vi "get data dimensions.vi"(8 "error in":errorcluster, 10 "# of groups":i32, 11 "Data (Dictionary)":T1[](array[typedef])) -> (0 "error out":errorcluster, 3 "data dimensions":i32[](array[numeric]))   [LabVIEW 2016]
uses:
  <userlib>/LevyLab/LV to ITX/Data/Typedefs/Dictionary--cluster.ctl
  <userlib>/LevyLab/LV to ITX/Data/Data.lvclass
panel:
  out "# groups (itx files)":i32
  out "# channels per file":i32
  out "# data pts per channel":dbl
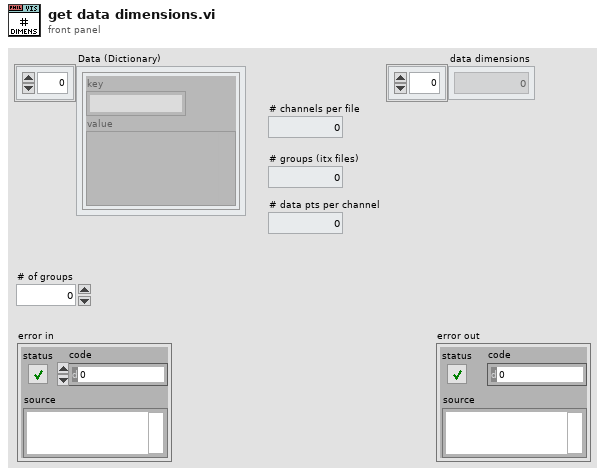
[diagram p1: front panel]
types:
  T1 = typedef "Data.lvclass/Dictionary--cluster.ctl" = cluster{"key":string, "value":variant}
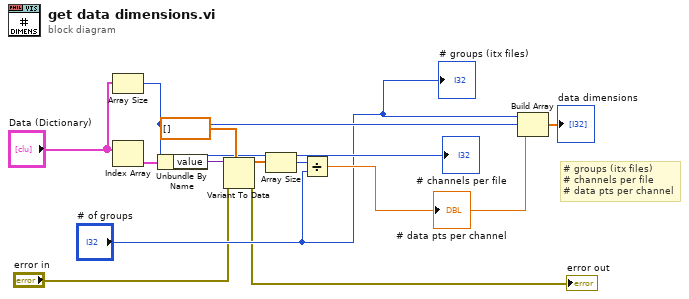
[diagram p0: block diagram]
diagram:
  # "# groups (itx files)\n# channels per file\n# data pts per channel"
  n1 = Array Size(array="Data (Dictionary)") -> (size(s)=w5:i32)
  "# channels per file" <- w5
  n2 = Index Array(array="Data (Dictionary)") -> (element=w8:T1)  [unwired: 1 in]
  n3 = Unbundle By Name(w8) -> ("value"=w9:variant)
  n4 = Variant To Data(error in="error in", type=dbl[] [], Variant=w9) -> (data=w11:dbl[], error out=→"error out":errorcluster)
  n5 = Array Size(array=w11) -> (size(s)=w12:i32)
  n6 = Divide(x=w12, y="# of groups") -> (x/y=w6:dbl)
  "# data pts per channel" <- w6
  n7 = Build Array("# of groups", w5, w6) -> (→"data dimensions":dbl[])
  "# groups (itx files)" <- "# of groups"
